vi "Append Refs.vi"(9 "Rename":string, 10 "Name":string) -> (1 "Post":string, 2 "Pre":string)   [LabVIEW 2025, in "_Rename.lvlib" / "_Rename.lvclass"]
uses:
  _Rename.lvclass
  _Rename.lvclass/_Rename.ctl
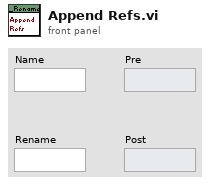
[diagram p1: front panel]
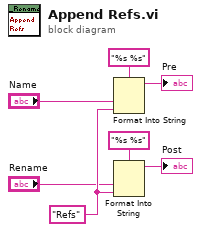
[diagram p0: block diagram]
diagram:
  w4 = "Refs" ("input 6")
  n1 = Format Into String(format string="%s %s", "Name", w4) -> (resulting string=→"Pre":string)  [unwired: 2 in, 1 out]
  n2 = Format Into String(format string="%s %s", "Rename", w4) -> (resulting string=→"Post":string)  [unwired: 2 in, 1 out]
